vi "Dispose.vi"(8 "error in (no error)":errorcluster, 11 "WebView2 Control in":refnum<class "WebView2 Control.lvclass">) -> (0 "error out":errorcluster)   [LabVIEW 2020, in "WebView2.lvlib" / "WebView2 Control.lvclass"]
uses:
  WebView2 Control.lvclass
  WebView2 Control.lvclass/WebView2 Control.ctl
  C:/Users/Simon/Documents/GitHub/LV-WebView2/Source/Libs/Microsoft.Web.WebView2.Core.dll
  Libs/Microsoft.Web.WebView2.Core.dll
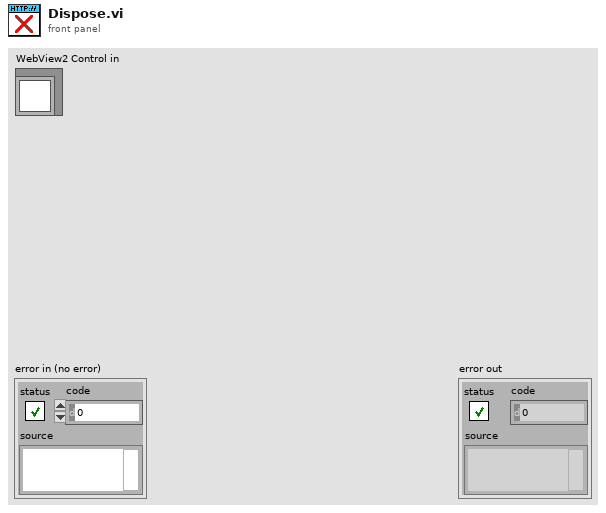
[diagram p1: front panel]
types:
  T1 = typedef "WebView2.lvlib/WebView2 Control.lvclass/Events.ctl" = cluster{"Navigation Complete Event":refnum<user-event>, "Source Changed Event":refnum<user-event>, "Document Title Changed Event":refnum<user-event>, "Status Bar Text Changed":refnum<user-event>, "Web Message Received":refnum<user-event>, "Window Close Requested":refnum<user-event>, "DOM Loaded":refnum<user-event>, "Navigation Started Event":refnum<user-event>}
  T2 = typedef "WebView2.lvlib/WebView2 Control.lvclass/Res.ctl" = cluster{"WebView2":refnum<k24>, "Webview2 Core":refnum<k24>, "event callback":refnum<k27>, "Environment":refnum<k24>}
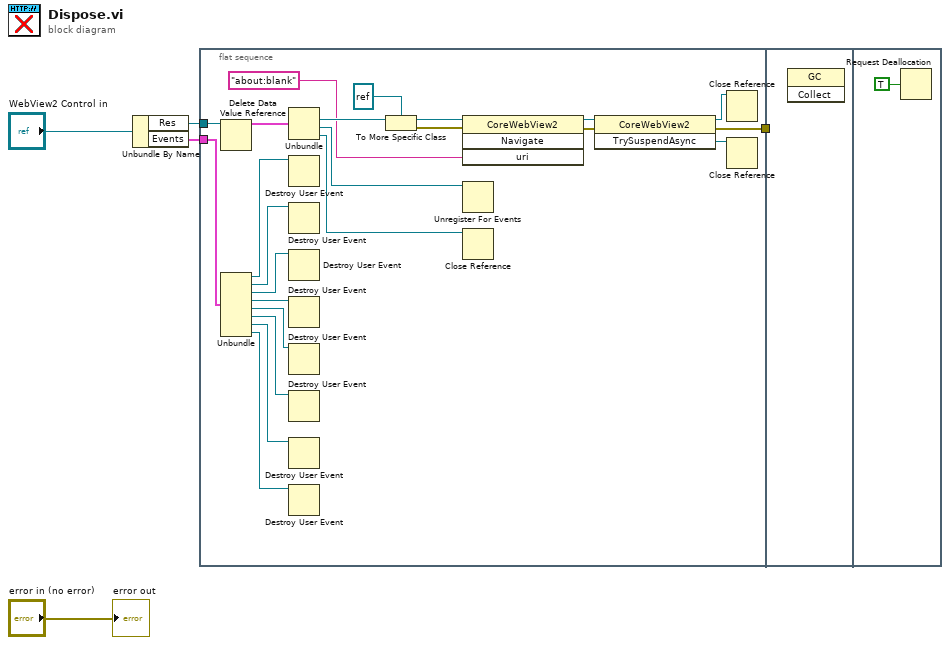
[diagram p0: block diagram]
diagram:
  n1 = Unbundle By Name("WebView2 Control in") -> ("Res"=w3:refnum<data-value>, "Events"=w2:T1)
  n2 = flat-sequence {
    tunnel: w3 -> [w10]
    tunnel: w2 -> [w28]
    tunnel: [w6] -> w1
    tunnel: w1 -> [_]
    frame #0 {
      n3 = Delete Data Value Reference(data value reference=w10) -> (data value=w11:T2)  [unwired: 1 in, 1 out]
      n4 = Unbundle(w28) -> ("Navigation Complete Event"=w27:refnum<user-event>, "Source Changed Event"=w26:refnum<user-event>, "Document Title Changed Event"=w25:refnum<user-event>, "Status Bar Text Changed"=w24:refnum<user-event>, "Web Message Received"=w23:refnum<user-event>, "Window Close Requested"=w22:refnum<user-event>, "DOM Loaded"=w21:refnum<user-event>, "Navigation Started Event"=w20:refnum<user-event>)
      n5 = Unbundle(w11) -> ("Webview2 Core"=w13:refnum<k24>, "event callback"=w19:refnum<k27>, "Environment"=w18:refnum<k24>)  [unwired: 1 out]
      n6 = Destroy User Event(user event=w27) -> ()  [unwired: 1 in, 1 out]
      n7 = Destroy User Event(user event=w26) -> ()  [unwired: 1 in, 1 out]
      n8 = Destroy User Event(user event=w25) -> ()  [unwired: 1 in, 1 out]
      n9 = Destroy User Event(user event=w24) -> ()  [unwired: 1 in, 1 out]
      n10 = Destroy User Event(user event=w23) -> ()  [unwired: 1 in, 1 out]
      n11 = Destroy User Event(user event=w22) -> ()  [unwired: 1 in, 1 out]
      n12 = Destroy User Event(user event=w21) -> ()  [unwired: 1 in, 1 out]
      n13 = Destroy User Event(user event=w20) -> ()  [unwired: 1 in, 1 out]
      n14 = To More Specific Class(target class=refnum<k24> refnum ("Webview2 Core"), reference=w13) -> (specific class reference=w9:refnum<k24>, error out=w7:errorcluster)  [unwired: 1 in]
      n15 = invoke class="CoreWebView2" method="Navigate"(reference=w9, error in=w7, "uri"="about:blank") -> (reference out=w16:refnum<k24>, error out=w17:errorcluster)  [unwired: 1 in, 2 out]
      n16 = Unregister For Events(event registration refnum=w19) -> ()  [unwired: 1 in, 1 out]
      n17 = Close Reference(reference=w18) -> ()  [unwired: 1 in, 1 out]
      n18 = invoke class="CoreWebView2" method="TrySuspendAsync"(reference=w16, error in=w17) -> (reference out=w14:refnum<k24>, error out=w6:errorcluster, "TrySuspendAsync"=w15:refnum<k24>)  [unwired: 1 in]
      n19 = Close Reference(reference=w14) -> ()  [unwired: 1 in, 1 out]
      n20 = Close Reference(reference=w15) -> ()  [unwired: 1 in, 1 out]
    }
    frame #1 {
      n21 = invoke class="GC" method="Collect"() -> ()  [unwired: 3 in, 3 out]
    }
    frame #2 {
      n22 = Request Deallocation(TRUE ("flag")) -> ()
    }
  }
  "error out" <- "error in (no error)"
